vi "ILABW_IsLoaded.vi"(3 "name":string) -> (0 "status":string)   [LabVIEW 2012]
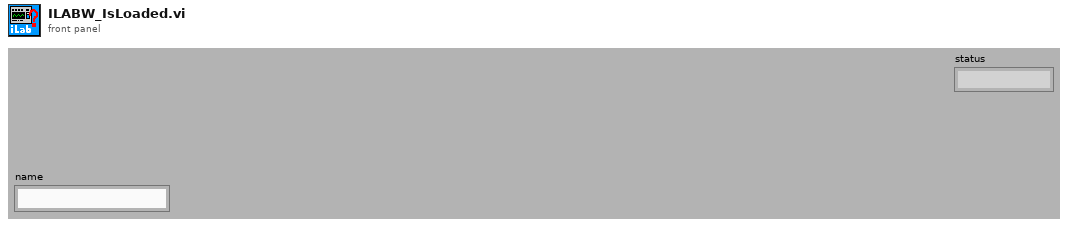
[diagram p1: front panel]
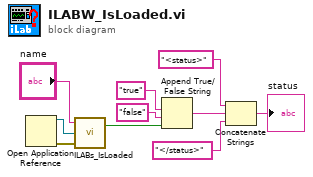
[diagram p0: block diagram]
diagram:
  n1 = Open Application Reference() -> (0:w10:errorcluster, 3:w9:refnum<vi>)  [unwired: 1 in, 3 out]
  n2 = call "ILABs_IsLoaded.vi"("error in (no error)"=w10, "appRef"=w9, "name"="name") -> ("status"=w7:bool)  [unwired: 1 out]
  n3 = Append True/False String(1:w7, 2:"false" ("false string"), 3:"true" ("true string")) -> (0:w2:string)  [unwired: 1 in]
  n4 = Concatenate Strings("<status>" ("string"), w2, "</status>" ("string")) -> (→"status":string)
